vi "determine_R_v07.vi"(0 "Pulse Data in (pA)":waveform(dbl)[](graph), 1 "memtest":T2={"Samples to Read"=2000, "Rate (Hz)"=20000.0, "Amplitude (mV/pA)"=10.0, "Offset (mV/pA)"=0.0, "Frequency (Hz)"=10.0, "duty cycle (%)"=50.0, "phase"=0.0} {"phase" format="%.2p"; "duty cycle (%)" format="%0.2f"}, 2 "replicates":i32=5, 3 "error in":errorcluster, 4 "Noise Data in (pA)":waveform(dbl)[](graph)) -> (6 "Power Spectrum":dbl[](graph), 7 "avg peak height":dbl, 8 "cell quality bad":bool, 9 "cell stats":T1 {"STD" format="%010.2f"; "Variance" format="%010.2f"; "Rt (MOhms)" format="%010.2f"; "tau (ms)" format="%08.2g"; "Cm (pF)" format="%08.2f"; "Ra (MOhms)" format="%010.2f"; "Rm (MOhms)" format="%010.2f"; "Ihold (pA)" format="%010.2f"}, 10 "error out":errorcluster)   [LabVIEW 2019]
uses:
  controls/memtest_def.ctl
  wc_protocol_v1.003 Folder/whole_cell_protocol/Controls/cell_stats-v02.ctl
  <vilib>/Analysis/2dsp.llb/Power Spectrum (DBL).vi
  <vilib>/Analysis/baseanly.llb/Mean (DBL).vi
  <vilib>/Analysis/8numeric.llb/1D Numeric Integration.vi
  <vilib>/Analysis/NI_AALBase.lvlib
  <vilib>/Analysis/NI_AALPro.lvlib
panel:
  out "Variance":dbl
  out "STD":dbl
  out "C (pF)":dbl
  out "Q (pA * s)":dbl format="%0.4f"
  out "transient":dbl[](graph)
  in  "fraction for Q":dbl=0.05
  out "t_stimOn":dbl
  out "Rm (MOhms)":dbl
  out "Ra (MOhms)":dbl
  out "peak value (pA)":dbl
  out "peak time (samples)":i32
  in  "peakOffset (samples)":i32=2
  out "Waveform Graph":dbl[](graph)
  out "first mean":dbl format="%0.2f"
  out "duration 2":dbl
  out "t_startFirst":dbl
  out "t_startSecond":dbl
  out "duration 1":dbl
  out "t_stimOff":dbl
  in  "fractionToSample":dbl=0.1
  out "R_total (MOhms)":dbl format="%#_13g"
  out "holding current out (pA)":dbl format="%#_13g"
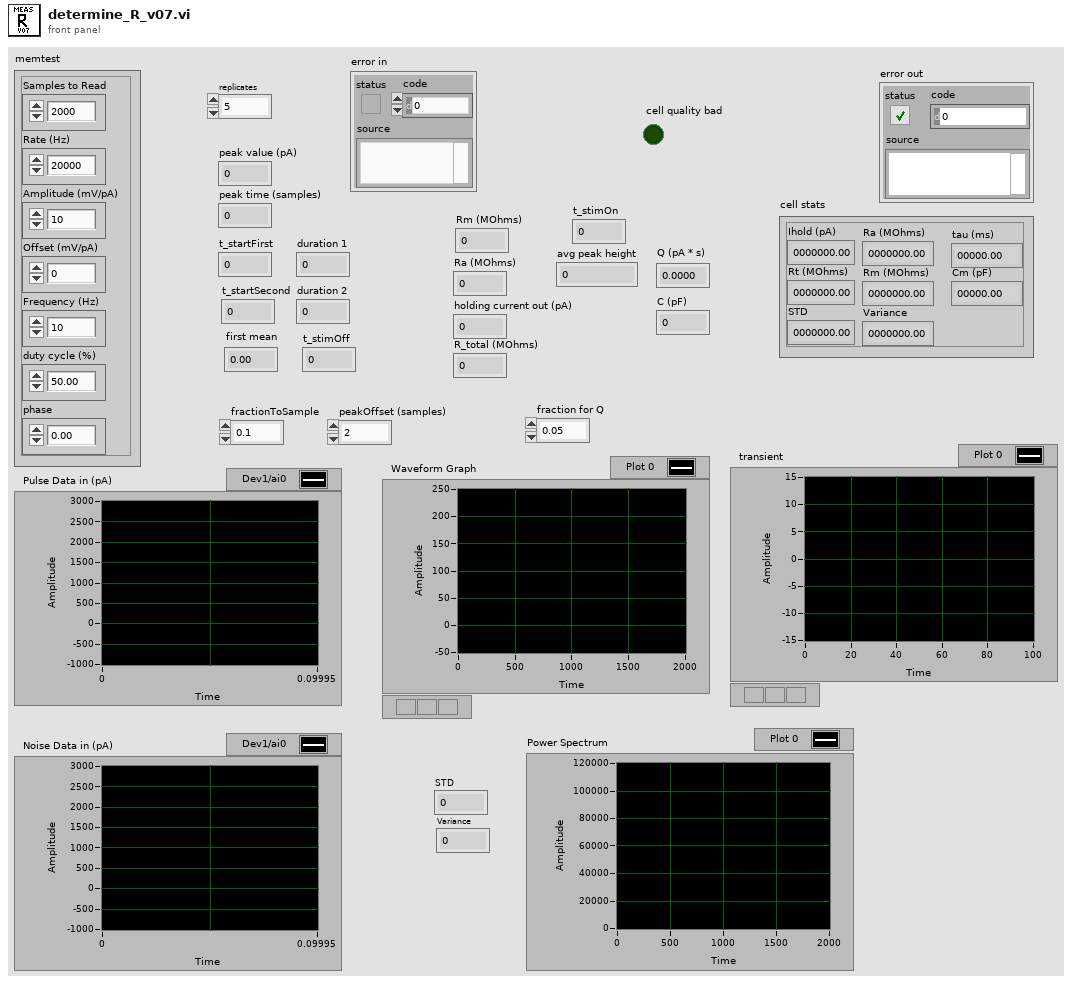
[diagram p1: front panel]
types:
  T1 = typedef "cell_stats-v02.ctl" = cluster{"Ihold (pA)":dbl, "Rm (MOhms)":dbl, "Ra (MOhms)":dbl, "Cm (pF)":dbl, "tau (ms)":dbl, "Rt (MOhms)":dbl, "Variance":dbl, "STD":dbl}
  T2 = typedef "memtest_def.ctl" = cluster{"Samples to Read":i32, "Rate (Hz)":dbl, "Amplitude (mV/pA)":dbl, "Offset (mV/pA)":dbl, "Frequency (Hz)":dbl, "duty cycle (%)":dbl, "phase":dbl}
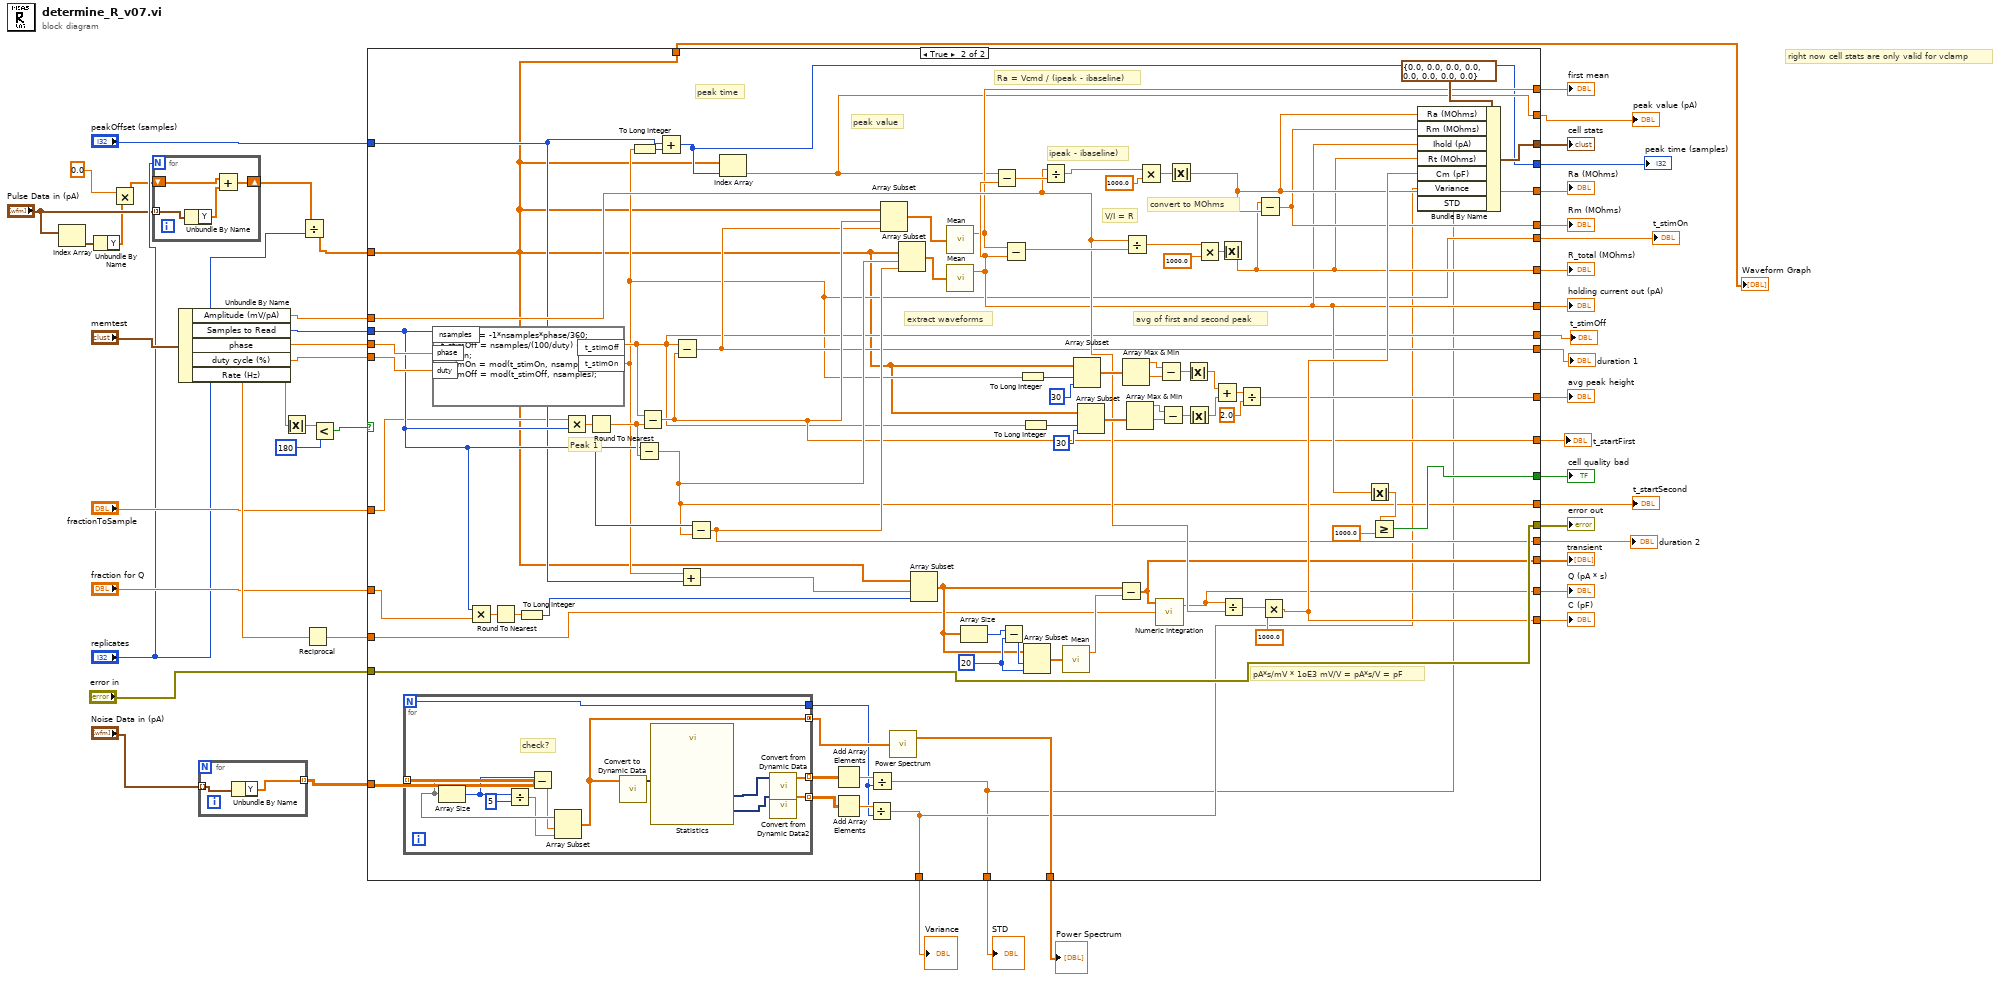
[diagram p0: block diagram]
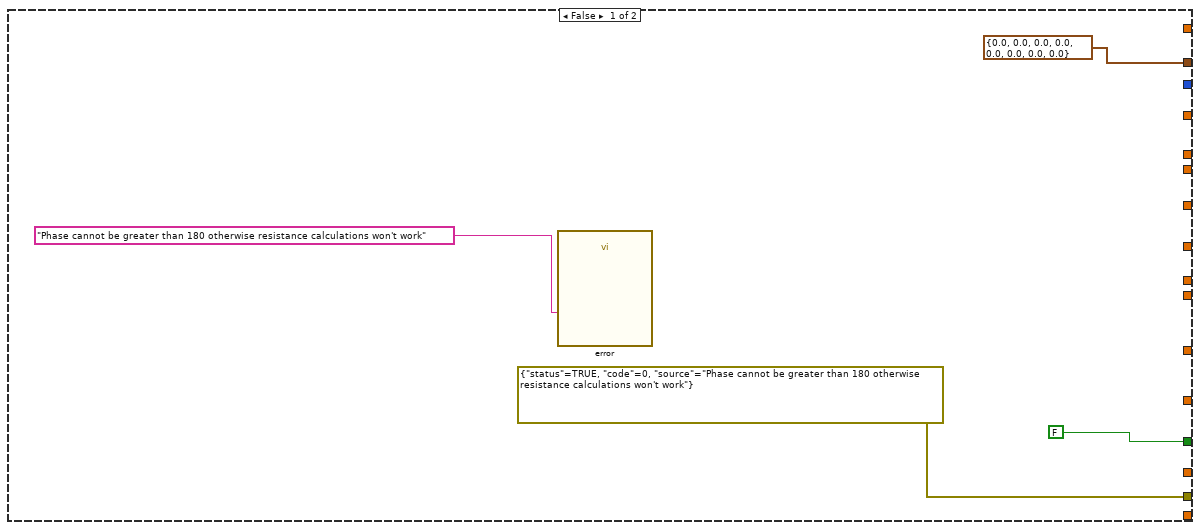
[diagram p2: hidden frame]
diagram:
  # "right now cell stats are only valid for vclamp"
  n1 = Index Array(array="Pulse Data in (pA)") -> (element=w5:waveform(dbl))  [unwired: 1 in]
  n2 = Unbundle By Name(w5) -> ("Y"=w3:dbl[])
  n3 = Multiply(x=0.0 ("y"), y=w3) -> (x*y=w2:dbl[])
  n4 = for {
    N: "replicates" -> [_]
    tunnel: "Pulse Data in (pA)" -> [w50] mode=indexing
    shift-right: [w52] -> w7
    shift-left: w2 -> [w51]
    n5 = Unbundle By Name(w50) -> ("Y"=w49:dbl[])
    n6 = Add(x=w51, y=w49) -> (x+y=w52:dbl[])
  }
  n7 = Unbundle By Name("memtest") -> ("Amplitude (mV/pA)"=w48:dbl, "Samples to Read"=w43:i32, "phase"=w40:dbl, "duty cycle (%)"=w47:dbl, "Rate (Hz)"=w38:dbl)
  n8 = for {
    tunnel: "Noise Data in (pA)" -> [w54] mode=indexing
    tunnel: [w53] -> w11 mode=indexing
    n9 = Unbundle By Name(w54) -> ("Y"=w53:dbl[])
  }
  n10 = Absolute Value(x=w40) -> (abs(x)=w44:dbl)
  n11 = Divide(x=w7, y="replicates") -> (x/y=w13:dbl[])
  n12 = Reciprocal(x=w38) -> (1/x=w37:dbl)
  n13 = Less?(x=w44, y=180) -> (x < y?=w45:bool)
  n14 = case shown="True" w45 {
    tunnel: w48 -> [_ w94]
    tunnel: w40 -> [_ w133]
    tunnel: w47 -> [_ w132]
    tunnel: w43 -> [_ w107]
    tunnel: [errorcluster {"status"=TRUE, "code"=0, "source"="Phase cannot be greater than 180 otherwise resistance calculations won't work"} ("error constant") w87] -> w41
    tunnel: [T1 {"Ihold (pA)"=0.0, "Rm (MOhms)"=0.0, "Ra (MOhms)"=0.0, "Cm (pF)"=0.0, "tau (ms)"=0.0, "Rt (MOhms)"=0.0, "Variance"=0.0, "STD"=0.0} ("cell stats 2") w125] -> w39
    tunnel: w37 -> [_ w98]
    tunnel: [FALSE w91] -> w36
    tunnel: "peakOffset (samples)" -> [_ w90]
    tunnel: w13 -> [_ w69]
    tunnel: "fractionToSample" -> [_ w89]
    tunnel: "fraction for Q" -> [_ w88]
    tunnel: "error in" -> [_ w87]
    tunnel: [_ w86] -> w31
    tunnel: [_ w85] -> w30
    tunnel: [_ w84] -> w29
    tunnel: [_ w83] -> w28
    tunnel: [_ w82] -> w27
    tunnel: [_ w81] -> w26
    tunnel: [_ w80] -> w25
    tunnel: [_ w79] -> w24
    tunnel: [_ w78] -> w23
    tunnel: [_ w77] -> w22
    tunnel: [_ w76] -> w21
    tunnel: [_ w75] -> w20
    tunnel: [_ w74] -> w19
    tunnel: [_ w73] -> w18
    tunnel: [_ w72] -> w17
    tunnel: [_ w71] -> w16
    tunnel: [_ w70] -> w15
    tunnel: [_ w69] -> w14
    tunnel: w11 -> [_ w68]
    tunnel: [_ w66] -> w10
    tunnel: [_ w60] -> w9
    tunnel: [_ w59] -> w8
    frame False {
      n15 = call "error"("Message"="Phase cannot be greater than 180 otherwise resistance calculations won't work" ("source")) -> ()  [unwired: 9 in, 2 out]
    }
    frame True {
      w102 = 20 ("y")
      # "pA*s/mV * 1oE3 mV/V = pA*s/V = pF"
      # "avg of first and second peak"
      # "ipeak - ibaseline)"
      # "Ra = Vcmd / (ipeak - ibaseline)"
      # "peak value"
      # "peak time"
      # "V/I = R"
      # "convert to MOhms"
      # "extract waveforms"
      # "Peak 1"
      n16 = for {
        N -> [w152]
        tunnel: w68 -> [w147] mode=indexing
        tunnel: [w152] -> w61
        tunnel: [w146] -> w67 mode=concatenating
        tunnel: [w150] -> w65 mode=indexing
        tunnel: [w148] -> w64 mode=indexing
        # "check?"
        n17 = Array Size(array=w147) -> (size(s)=w145:i32)
        n18 = Divide(x=w145, y=5) -> (x/y=w142:dbl)
        n19 = Subtract(x=w145, y=w142) -> (x-y=w143:dbl)
        n20 = Array Subset(array=w147, index=w143, length=w142) -> (w146:dbl[])
        n21 = call "Convert to Dynamic Data"("Array"=w146) -> ("Dynamic Data Type"=w153:dynamicdata)  [unwired: 3 in]
        n22 = call "Statistics"("Signals"=w153) -> ("Variance"=w149:dynamicdata, "Standard Dev"=w151:dynamicdata)  [unwired: 24 in, 1 out]
        n23 = call "Convert from Dynamic Data"("Dynamic Data Type"=w151) -> ("Array"=w150:dbl[])  [unwired: 3 in]
        n24 = call "Convert from Dynamic Data2"("Dynamic Data Type"=w149) -> ("Array"=w148:dbl[])  [unwired: 3 in]
      }
      n25 = formula code="t_stimOn = -1*nsamples*phase/360;\nt_stimOff = nsamples/(100/duty) +t_stimOn;\nt_stimOn = mod(t_stimOn, nsamples);\nt_stimOff = mod(t_stimOff, nsamples);"("nsamples"=w107, "phase"=w133, "duty"=w132) -> ("t_stimOff"=w73:dbl, "t_stimOn"=w72:dbl)
      n26 = Multiply(x=w107, y=w88) -> (x*y=w108:dbl)
      n27 = Round To Nearest(number=w108) -> (nearest integer value=w106:dbl)
      n28 = To Long Integer(number=w106) -> (32bit integer=w105:i32)
      n29 = Multiply(x=w89, y=w107) -> (x*y=w141:dbl)
      n30 = Round To Nearest(number=w141) -> (nearest integer value=w140:dbl)
      n31 = To Long Integer(number=w72) -> (32bit integer=w131:i32)
      n32 = Subtract(x=w107, y=w140) -> (x-y=w76:dbl)
      n33 = Subtract(x=w73, y=w140) -> (x-y=w75:dbl)
      n34 = Add(x=w90, y=w131) -> (x+y=w70:i32)
      n35 = Subtract(x=w73, y=w75) -> (x-y=w74:dbl)
      n36 = Add(x=w72, y=w90) -> (x+y=w96:dbl)
      n37 = Subtract(x=w107, y=w76) -> (x-y=w77:dbl)
      n38 = Index Array(array=w69, index=w70) -> (element=w71:dbl)
      n39 = Add Array Elements(numeric array=w65) -> (sum=w63:dbl)
      n40 = Add Array Elements(numeric array=w64) -> (sum=w62:dbl)
      n41 = Divide(x=w62, y=w61) -> (x/y=w60:dbl)
      n42 = Divide(x=w63, y=w61) -> (x/y=w59:dbl)
      n43 = Array Subset(array=w69, index=w75, length=w74) -> (w139:dbl[])
      n44 = call-poly <vilib>:"Power Spectrum.vi"("X"=w67) -> ("Power Spectrum"=w66:dbl[])  [unwired: 1 out]
      n45 = Array Subset(array=w69, index=w76, length=w77) -> (w138:dbl[])
      n46 = Array Subset(array=w69, index=w96, length=w105) -> (w99:dbl[])
      n47 = call-poly <vilib>:"Mean.vi"("X"=w139) -> ("mean"=w78:dbl)  [unwired: 1 out]
      n48 = call-poly <vilib>:"Mean.vi"("X"=w138) -> ("mean"=w79:dbl)  [unwired: 1 out]
      n49 = Array Size(array=w99) -> (size(s)=w104:i32)
      n50 = Subtract(x=w71, y=w79) -> (x-y=w130:dbl)
      n51 = Subtract(x=w104, y=w102) -> (x-y=w103:i32)
      n52 = Subtract(x=w78, y=w79) -> (x-y=w137:dbl)
      n53 = To Long Integer(number=w72) -> (32bit integer=w110:i32)
      n54 = To Long Integer(number=w73) -> (32bit integer=w109:i32)
      n55 = Array Subset(array=w99, index=w103, length=w102) -> (w101:dbl[])
      n56 = Divide(x=w94, y=w130) -> (x/y=w129:dbl)
      n57 = call-poly <vilib>:"Mean.vi"("X"=w101) -> ("mean"=w100:dbl)  [unwired: 1 out]
      n58 = Array Subset(array=w69, index=w110, length=30) -> (w123:dbl[])
      n59 = Array Subset(array=w69, index=w109, length=30) -> (w121:dbl[])
      n60 = Subtract(x=w99, y=w100) -> (x-y=w84:dbl[])
      n61 = Array Max & Min(array=w123) -> (max value=w120:dbl, min value=w119:dbl)  [unwired: 2 out]
      n62 = Divide(x=w94, y=w137) -> (x/y=w135:dbl)
      n63 = Array Max & Min(array=w121) -> (max value=w118:dbl, min value=w117:dbl)  [unwired: 2 out]
      n64 = Multiply(x=w129, y=1000.0) -> (x*y=w127:dbl)
      n65 = call-poly <vilib>:"Numeric Integration.vi"("dt"=w98, "Input Array"=w84) -> ("result"=w85:dbl)  [unwired: 1 in, 1 out]
      n66 = Subtract(x=w120, y=w119) -> (x-y=w116:dbl)
      n67 = Subtract(x=w118, y=w117) -> (x-y=w115:dbl)
      n68 = Absolute Value(x=w127) -> (abs(x)=w82:dbl)
      n69 = Absolute Value(x=w116) -> (abs(x)=w114:dbl)
      n70 = Absolute Value(x=w115) -> (abs(x)=w113:dbl)
      n71 = Multiply(x=w135, y=1000.0) -> (x*y=w136:dbl)
      n72 = Add(x=w114, y=w113) -> (x+y=w112:dbl)
      n73 = Absolute Value(x=w136) -> (abs(x)=w80:dbl)
      n74 = Divide(x=w85, y=w94) -> (x/y=w95:dbl)
      n75 = Divide(x=w112, y=2.0) -> (x/y=w83:dbl)
      n76 = Subtract(x=w80, y=w82) -> (x-y=w81:dbl)
      n77 = Multiply(x=w95, y=1000.0) -> (x*y=w86:dbl)
      n78 = Absolute Value(x=w79) -> (abs(x)=w92:dbl)
      n79 = Greater Or Equal?(x=w92, y=1000.0) -> (x >= y?=w91:bool)
      n80 = Bundle By Name(cluster=T1 {"Ihold (pA)"=0.0, "Rm (MOhms)"=0.0, "Ra (MOhms)"=0.0, "Cm (pF)"=0.0, "tau (ms)"=0.0, "Rt (MOhms)"=0.0, "Variance"=0.0, "STD"=0.0} ("cell stats 2"), "Ra (MOhms)"=w82, "Rm (MOhms)"=w81, "Ihold (pA)"=w79, "Rt (MOhms)"=w80, "Cm (pF)"=w86, "Variance"=w60, "STD"=w59) -> (w125:T1)
    }
  }
  "error out" <- w41
  "cell stats" <- w39
  "cell quality bad" <- w36
  "C (pF)" <- w31
  "Q (pA * s)" <- w30
  "transient" <- w29
  "avg peak height" <- w28
  "holding current out (pA)" <- w24
  "R_total (MOhms)" <- w25
  "Ra (MOhms)" <- w27
  "Rm (MOhms)" <- w26
  "first mean" <- w23
  "duration 2" <- w22
  "t_startSecond" <- w21
  "t_startFirst" <- w20
  "duration 1" <- w19
  "t_stimOff" <- w18
  "t_stimOn" <- w17
  "peak value (pA)" <- w16
  "peak time (samples)" <- w15
  "Waveform Graph" <- w14
  "Power Spectrum" <- w10
  "STD" <- w8
  "Variance" <- w9
